vi "MIMO Tx Streaming Multi-Channel (Host).vi"() -> ()   [LabVIEW 2013]
doc: "This template is for the Simple NI-USRP Streaming design, a design that shows the basics of streaming data from an NI 294x/295x device. Refer to the block diagram for more information about how to use this template."
uses:
  <vilib>/userdefined/Silver/nirio_resource_slv.ctl
  SubVIs/Start Trigger.ctl
  <vilib>/Utility/error.llb/DialogType.ctl
  SubVIs/Configure Signal (Level).vi
  SubVIs/Write Tx Data (I16 multi).vi
panel:
  out "Output Waveform":waveform(dbl)[](graph)
  out "generating":bool caption="Generating"
  in  "tone frequency":dbl=100000.0 caption="Tone Frequency" format="%#.3pHz"
  in  "number of samples is finite":bool
  in  "reference level rf 1":dbl caption="Reference Level" format="%#_gdBm"
  in  "reference level rf 0":dbl caption="Reference Level" format="%#_gdBm"
  in  "lo frequency rf 1":dbl=-1.0 caption="LO Frequency" format="%#.3pHz"
  in  "lo frequency rf 0":dbl=-1.0 caption="LO Frequency" format="%#.3pHz"
  in  "frequency rf 1":dbl=2000000000.0 caption="Frequency" format="%#.3pHz"
  in  "frequency rf 0":dbl=2000000000.0 caption="Frequency" format="%#.3pHz"
  in  "antenna rf 1":string(combo)="TX1" caption="Active Antenna"
  in  "antenna rf 0":string(combo)="TX1" caption="Active Antenna"
  in  "enable rf 1":bool=TRUE
  in  "enable rf 0":bool=TRUE
  in  "USRP RIO devices":T1[](array[typedef])=["RIO0", "RIO1"] caption="USRP RIO Devices"
  in  "reference frequency source":string(combo)="REF IN" caption="Reference Frequency Source"
  in  "sample rate":dbl=10000000.0 caption="Sample Rate" format="%#.3pS/s"
  in  "start trigger":T2=enum."Immediate" caption="Start Trigger"
  in  "number of samples":u32=1000000 caption="Number of Samples"
  in  "stop":bool
  # "Multi-Channel MIMO Tx Streaming"
  # "This template is for the Simple NI-USRP Streaming design, a design that shows the basics of streaming data from an NI 294x/295x device. See the block diagram for more information on how to use this template."
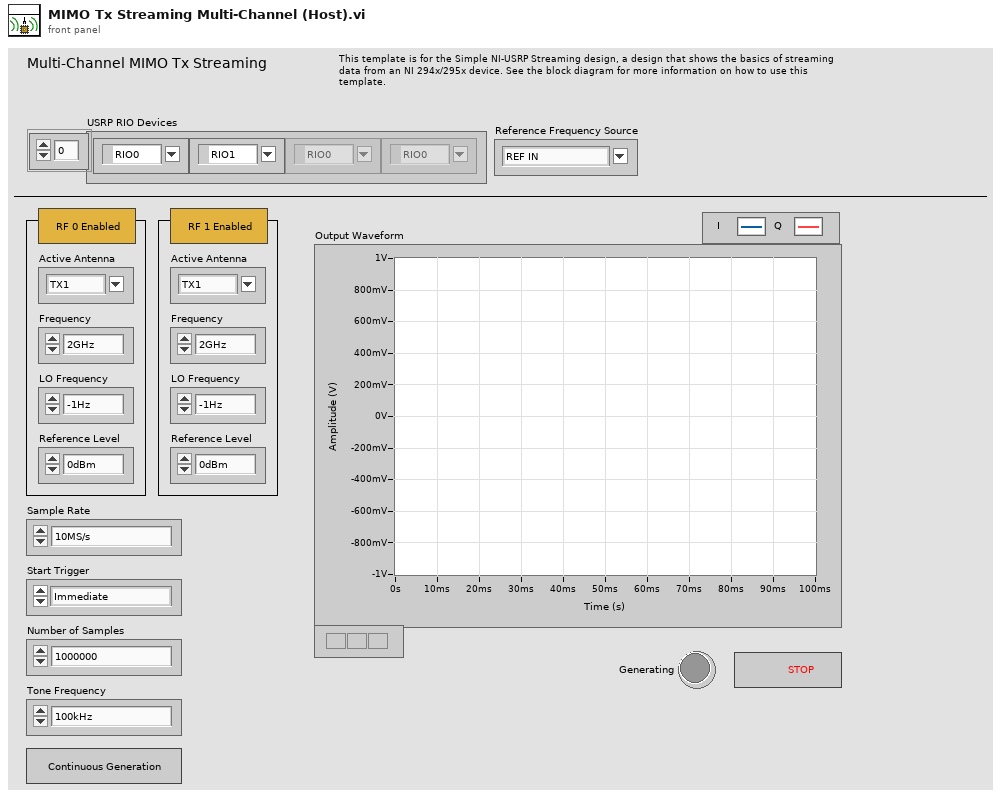
[diagram p1: front panel]
types:
  T1 = typedef "nirio_resource_slv.ctl" = tag
  T2 = typedef "Start Trigger.ctl" = enum8{"Software", "Digital Edge", "Rx Start Trigger", "Tx Start Trigger", "Immediate"}
  T3 = typedef "DialogType.ctl" = u16
  T4 = typedef "niUsrpRio Config v1 Host.lvlib/niUsrpRio Session.ctl" = cluster{"Global Settings Register Bus":T5, "Radio 0 Settings Register Bus":T5, "Rx NI-USRP session":refnum<k15>, "Tx NI-USRP session":refnum<k15>, "FPGA Interface":refnum<k20>, "RIO Interface Number":u32, "EEPROM Header":T6, "Device Data Header":T7, "EEPROM Characterization Header":T8, "Characterization Data":T9[], "Characterization Data Valid?":bool, "Radio 1 Settings Register Bus":T5, "Radio Settings Bus Semaphore":T11}
  T5 = typedef "niInstr Register Bus v0 Host.lvlib/Register Bus Session.ctl" = refnum<queue>
  T6 = typedef "niUsrpRio Config v1 Host.lvlib/EEPROM Header.ctl" = cluster{"Checksum":u32, "Product Code":u16, "Hardware Current Version":u16, "Hardware Oldest Compatible Version":u16, "EEPROM Map Current Version":u16, "EEPROM Map Oldest Compatible Version":u16, "User Password":string, "Pointer to Factory Header":u32, "Pointer to User Header":u32, "Recommended Interval":u16, "Number of Reserved Bytes":i32, "Number of Daughterboards":u8, "Daughterboard IDs":u16[], "Daughterboard Serial Numbers":string[]}
  T7 = typedef "niUsrpRio Config v1 Host.lvlib/EEPROM Device Data Header.ctl" = cluster{"Checksum":u32, "Number of Channels":u8, "Number of Gain Settings":u16[], "Pointer to Characterization Data":u32[], "Number of Reserved Bytes":i32, "Number of Frequencies":u16[]}
  T8 = typedef "niUsrpRio Config v1 Host.lvlib/EEPROM Characterization Header.ctl" = cluster{"Checksum":u32, "Date":timestamp, "Temperature":sgl, "Misc. Info":string, "Pointer to Device Data Header":u32, "Number of Reserved Bytes":i32}
  T9 = typedef "niUsrpRio Config v1 Host.lvlib/Characterization Data.ctl" = cluster{"Gains[dB]":dbl[], "Frequencies [Hz]":dbl[], "IQ Imbalance Table":T10[], "Measured Gains[dB]":dbl[][]}
  T10 = typedef "niUsrpRio Config v1 Host.lvlib/IQ Imbalance.ctl" = cluster{"Gain Imbalance [linear]":dbl, "Phase Imbalance [radians]":dbl, "Offset":cdb}
  T11 = typedef "Semaphore RefNum" = refnum<k1>
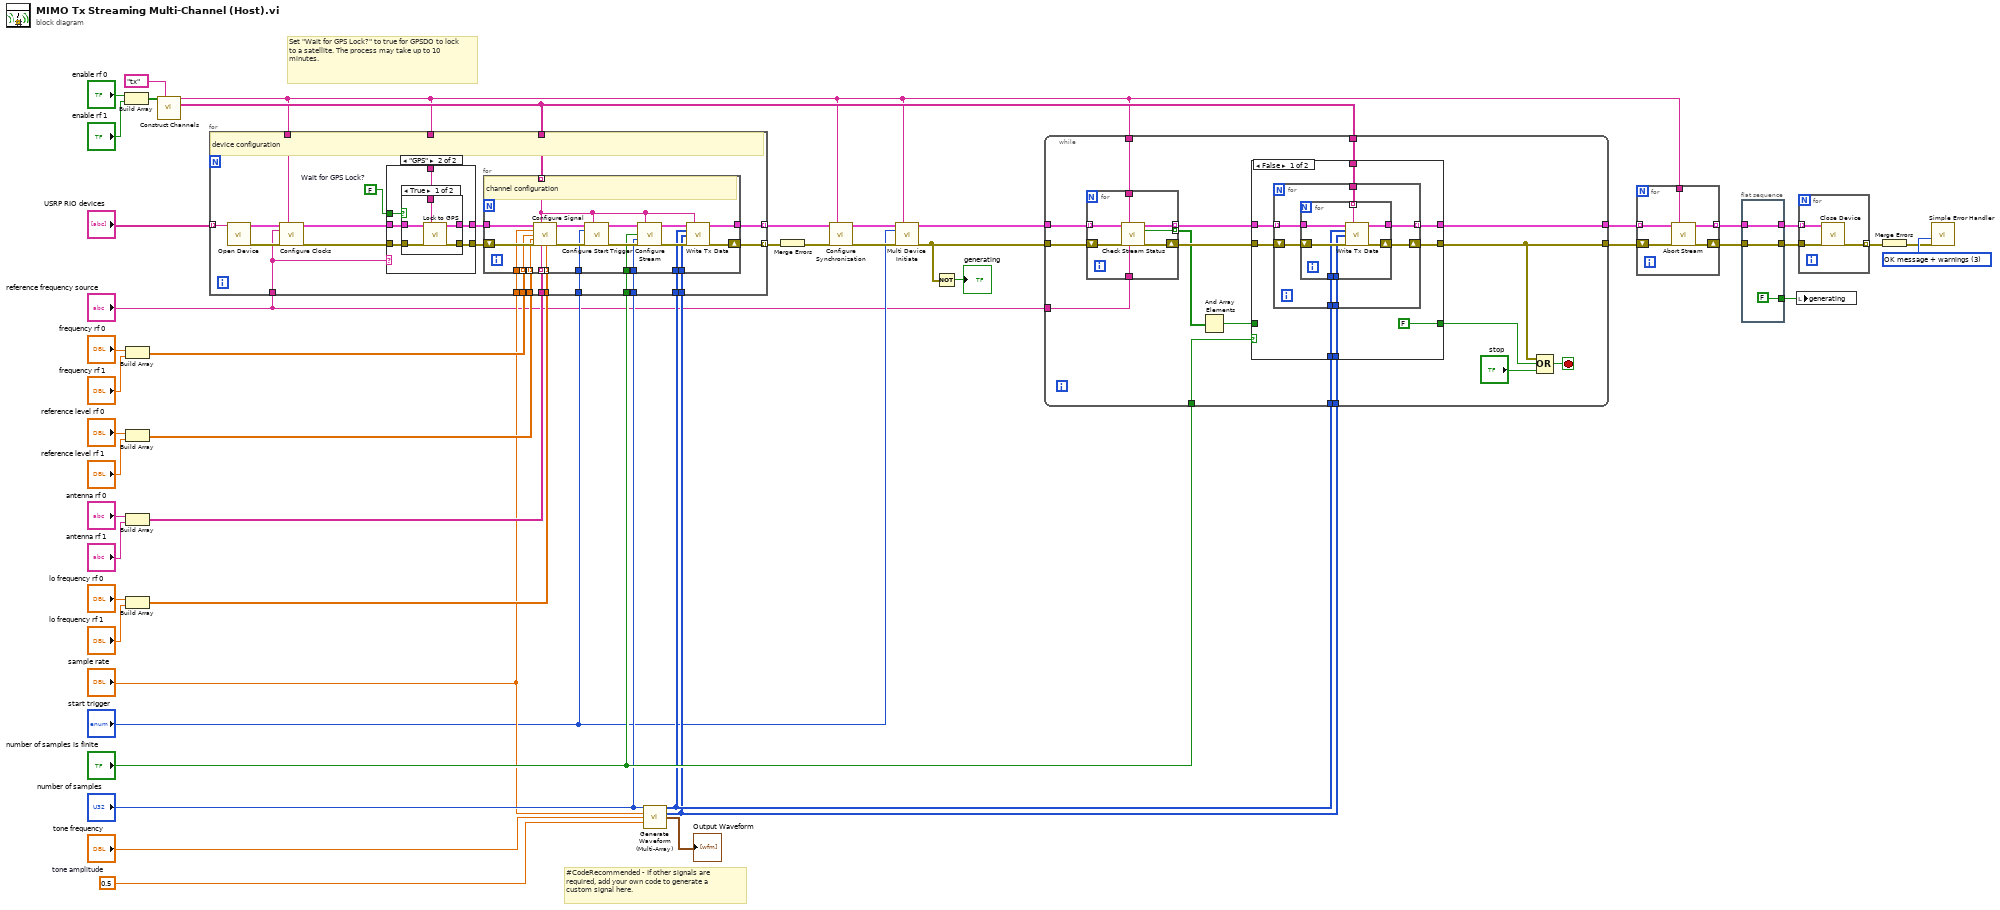
[diagram p0: block diagram]
diagram:
  w16 = 0.5  # tone amplitude
  w44 = T3 3 items=["no dialog", "OK message", "continue or stop message", "OK message + warnings", "continue/stop + warnings"] ("type of dialog (OK msg:1)")
  # "#CodeRecommended - If other signals are required, add your own code to generate a custom signal here."
  # "Set \"Wait for GPS Lock?\" to true for GPSDO to lock to a satellite. The process may take up to 10 minutes."
  n1 = Build Array("enable rf 0", "enable rf 1") -> (w33:bool[])
  n2 = Build Array("frequency rf 0", "frequency rf 1") -> (w23:dbl[])
  n3 = Build Array("reference level rf 0", "reference level rf 1") -> (w24:dbl[])
  n4 = Build Array("antenna rf 0", "antenna rf 1") -> (w32:string[])
  n5 = Build Array("lo frequency rf 0", "lo frequency rf 1") -> (w27:dbl[])
  n6 = call "Construct Channels.vi"("enabled channels"=w33, "scope"="tx") -> ("scope"=w2:string, "channels"=w21:string[])  [unwired: 12 in]
  n7 = call "Generate Waveform (Multi-Array).vi"("number of samples"="number of samples", "sample rate"="sample rate", "tone frequency"="tone frequency", "amplitude"=w16) -> ("I"=w14:i16[], "Q"=w13:i16[], "Waveform"=→"Output Waveform":waveform(dbl)[])  [unwired: 9 in]
  n8 = for {
    tunnel: [w71] -> w46 mode=indexing
    tunnel: [w70] -> w43 mode=indexing
    tunnel: "start trigger" -> [w69]
    tunnel: "number of samples" -> [w66]
    tunnel: "number of samples is finite" -> [w65]
    tunnel: "reference frequency source" -> [w51]
    tunnel: w27 -> [w64]
    tunnel: w23 -> [w63]
    tunnel: w24 -> [w62]
    tunnel: w21 -> [w61]
    tunnel: "sample rate" -> [w60]
    tunnel: "USRP RIO devices" -> [w59] mode=indexing
    tunnel: w32 -> [w58]
    tunnel: w2 -> [w57]
    tunnel: w2 -> [w50]
    tunnel: w13 -> [w49]
    tunnel: w14 -> [w48]
    w56 = FALSE  # Wait for GPS Lock?
    # "device configuration"
    n9 = call "Open Device.vi"("USRP RIO device"=w59) -> ("niUsrpRio Session (out)"=w68:T4, "error out"=w67:errorcluster)  [unwired: 13 in]
    n10 = call "Configure Clocks.vi"("niUsrpRio Session"=w68, "scope"=w57, "Reference Frequency Source"=w51, "error in"=w67) -> ("niUsrpRio Session (out)"=w53:T4, "error out"=w54:errorcluster)  [unwired: 10 in]
    n11 = case shown="\"GPS\"" w51 {
      tunnel: w53 -> [w73 w79]
      tunnel: [w73 w78] -> w52
      tunnel: [w72 w77] -> w55
      tunnel: w54 -> [w72 w76]
      tunnel: w50 -> [_ w75]
      tunnel: w56 -> [_ w74]
      frame Default {
      }
      frame "GPS" {
        n12 = case shown="True" w74 {
          tunnel: w79 -> [w81 w86]
          tunnel: [w84 w86] -> w78
          tunnel: [w83 w85] -> w77
          tunnel: w76 -> [w80 w85]
          tunnel: w75 -> [w82 _]
          frame True {
            n13 = call "Lock to GPS.vi"("niUsrpRio Session"=w81, "scope"=w82, "error in"=w80) -> ("niUsrpRio Session (out)"=w84:T4, "error out"=w83:errorcluster)  [unwired: 11 in]
          }
          frame False {
          }
        }
      }
    }
    n14 = for {
      tunnel: [w90] -> w70
      tunnel: w69 -> [w105]
      tunnel: w52 -> [w100]
      tunnel: w66 -> [w99]
      tunnel: w65 -> [w98]
      shift-right: [w92] -> w71
      shift-left: w55 -> [w101]
      tunnel: w61 -> [w89] mode=indexing
      tunnel: w64 -> [w97] mode=indexing
      tunnel: w63 -> [w96] mode=indexing
      tunnel: w62 -> [w95] mode=indexing
      tunnel: w60 -> [w94]
      tunnel: w58 -> [w93] mode=indexing
      tunnel: w49 -> [w88]
      tunnel: w48 -> [w87]
      # "channel configuration"
      n15 = call-poly "Configure Signal.vi"("niUsrpRio Session"=w100, "scope"=w89, "sample rate [S/s]"=w94, "frequency [Hz]"=w96, "level [dBm]"=w95, "error in"=w101, "Active Antenna"=w93, "LO frequency [Hz]"=w97) -> ("niUsrpRio Session (out)"=w103:T4, "error out"=w107:errorcluster)  [unwired: 1 in, 5 out]
      n16 = call "Configure Start Trigger.vi"("niUsrpRio Session"=w103, "scope"=w89, "start trigger"=w105, "error in"=w107) -> ("niUsrpRio Session (out)"=w102:T4, "error out"=w104:errorcluster)  [unwired: 10 in]
      n17 = call "Configure Stream.vi"("niUsrpRio Session"=w102, "scope"=w89, "number of samples is finite"=w98, "number of samples"=w99, "error in"=w104) -> ("niUsrpRio Session (out)"=w91:T4, "error out"=w106:errorcluster)  [unwired: 9 in]
      n18 = call-poly "Write Tx Data.vi"("niUsrpRio Session"=w91, "scope"=w89, "I"=w87, "Q"=w88, "error in"=w106) -> ("niUsrpRio Session (out)"=w90:T4, "error out"=w92:errorcluster)  [unwired: 9 in]
    }
  }
  n19 = Merge Errors(w46) -> (w39:errorcluster)
  n20 = call "Configure Synchronization.vi"("niUsrpRio Sessions"=w43, "scope"=w2, "error in"=w39) -> ("niUsrpRio Sessions (out)"=w5:T4[], "error out"=w47:errorcluster)  [unwired: 11 in]
  n21 = call "Multi Device Initiate.vi"("niUsrpRio Sessions"=w5, "scope"=w2, "start trigger"="start trigger", "error in"=w47) -> ("niUsrpRio Sessions (out)"=w3:T4[], "error out"=w4:errorcluster)  [unwired: 10 in]
  n22 = Not(x=w4) -> (.not. x?=→"generating":bool)
  n23 = while {
    tunnel: [w122] -> w42
    tunnel: [w121] -> w41
    tunnel: "number of samples is finite" -> [w112]
    tunnel: w21 -> [w120]
    tunnel: w14 -> [w119]
    tunnel: w13 -> [w118]
    tunnel: w4 -> [w116]
    tunnel: w3 -> [w117]
    tunnel: w2 -> [w109]
    tunnel: "reference frequency source" -> [w108]
    stop <- w124 stop-if-true
    # "Acquire and Fetch a waveform"
    n24 = for {
      tunnel: w117 -> [w156] mode=indexing
      tunnel: [w153] -> w115 mode=indexing
      tunnel: [w152] -> w113 mode=indexing
      shift-right: [w154] -> w114
      shift-left: w116 -> [w155]
      tunnel: w109 -> [w151]
      tunnel: w108 -> [w150]
      n25 = call "Check Stream Status.vi"("niUsrpRio Session"=w156, "scope"=w151, "error in"=w155, "reference frequency source"=w150) -> ("niUsrpRio Session (out)"=w153:T4, "done"=w152:bool, "error out"=w154:errorcluster)  [unwired: 9 in]
    }
    n26 = And Array Elements(Boolean array=w113) -> (logical AND=w111:bool)
    n27 = case shown="False" w112 {
      tunnel: [w132 w148] -> w122
      tunnel: [w131 w149] -> w121
      tunnel: w120 -> [w130 _]
      tunnel: w119 -> [w129 _]
      tunnel: w118 -> [w128 _]
      tunnel: w115 -> [w127 w148]
      tunnel: w114 -> [w126 w149]
      tunnel: [FALSE w147] -> w110
      tunnel: w111 -> [_ w147]
      frame False {
        n28 = for {
          tunnel: [w133] -> w132 mode=indexing
          tunnel: w127 -> [w137] mode=indexing
          tunnel: w130 -> [w138]
          shift-right: [w134] -> w131
          shift-left: w126 -> [w139]
          tunnel: w129 -> [w136]
          tunnel: w128 -> [w135]
          n29 = for {
            shift-right: [w145] -> w134
            shift-left: w139 -> [w146]
            tunnel: w138 -> [w143] mode=indexing
            tunnel: w137 -> [w144]
            tunnel: [w142] -> w133
            tunnel: w135 -> [w141]
            tunnel: w136 -> [w140]
            n30 = call-poly "Write Tx Data.vi"("niUsrpRio Session"=w144, "scope"=w143, "I"=w140, "Q"=w141, "error in"=w146) -> ("niUsrpRio Session (out)"=w142:T4, "error out"=w145:errorcluster)  [unwired: 9 in]
          }
        }
      }
      frame True {
      }
    }
    n31 = Compound Arithmetic op=OR(w121, w110, "stop") -> (w124:bool)
  }
  n32 = for {
    tunnel: w42 -> [w161] mode=indexing
    tunnel: [w160] -> w10 mode=indexing
    shift-right: [w158] -> w11
    shift-left: w41 -> [w159]
    tunnel: w2 -> [w157]
    n33 = call "Abort Stream.vi"("niUsrpRio Session"=w161, "scope"=w157, "error in"=w159) -> ("niUsrpRio Session (out)"=w160:T4, "error out"=w158:errorcluster)  [unwired: 11 in]
  }
  n34 = flat-sequence {
    tunnel: [w164] -> w9
    tunnel: w10 -> [w164]
    tunnel: [w163] -> w8
    tunnel: w11 -> [w163]
    tunnel: [FALSE ("Generating")] -> w7
    frame #0 {
    }
  }
  n35 = local write "generating"(w7) -> ()
  n36 = for {
    tunnel: [w167] -> w45 mode=indexing
    tunnel: w9 -> [w166] mode=indexing
    tunnel: w8 -> [w165]
    n37 = call "Close Device.vi"("niUsrpRio Session"=w166, "error in"=w165) -> ("error out"=w167:errorcluster)  [unwired: 13 in]
  }
  n38 = Merge Errors(w45) -> (w38:errorcluster)
  n39 = call <vilib>:"Simple Error Handler.vi"("type of dialog (OK msg:1)"=w44, "error in (no error)"=w38) -> ()  [unwired: 3 in, 5 out]
